vi "Q2.vi"() -> ()   [LabVIEW 2019]
uses:
  <vilib>/measure/matone.llb/Extract Multiple Tone Information N Chan.vi
  <vilib>/measure/NI_MAPro.lvlib
panel:
  in  "Boolean":bool
  out "Potência Ativa":i32
  out "multiple tone information":T1(array[cluster]) {"multiple tone information"."detected phase (deg)" format="%_6g"; "multiple tone information"."detected amplitude" format="%_6p"; "multiple tone information"."detected frequency" format="%_6p"}
  out "Waveform Graph":waveform(dbl)[](graph)
  in  "file path":path
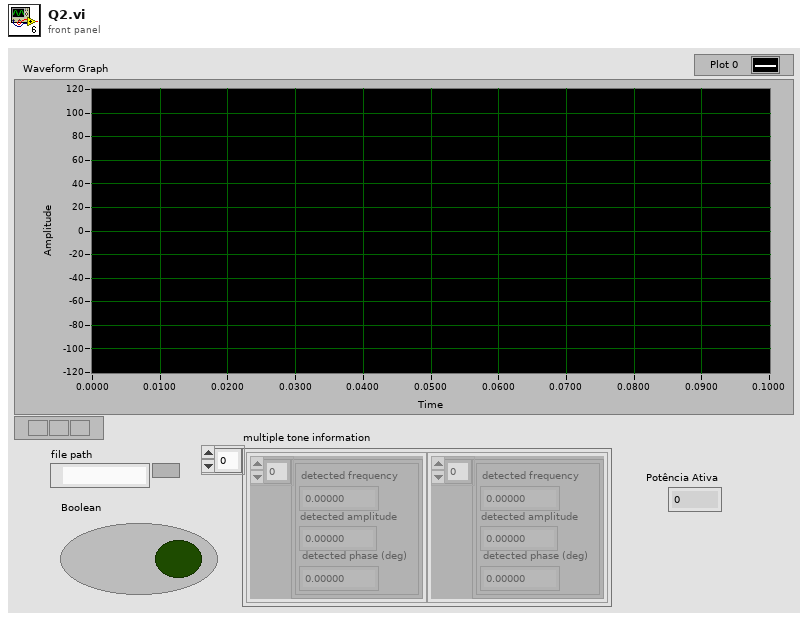
[diagram p1: front panel]
types:
  T1 = cluster{"multiple tone information":cluster{"detected frequency":dbl, "detected amplitude":dbl, "detected phase (deg)":dbl}[]}[]
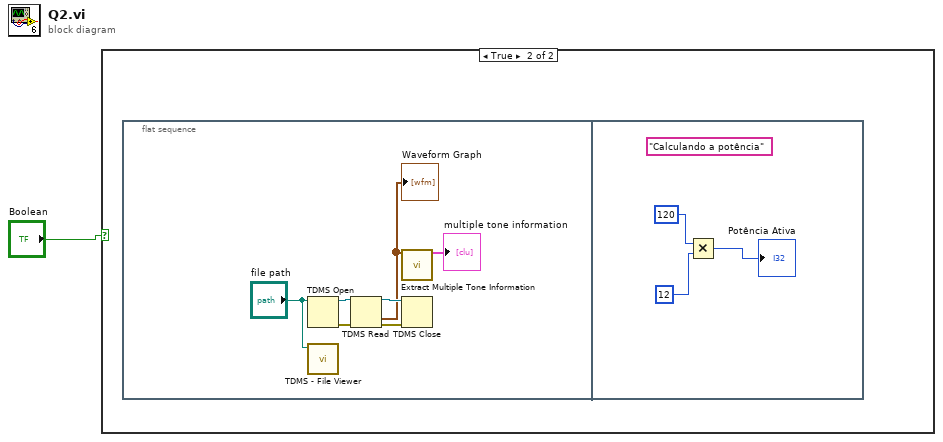
[diagram p0: block diagram]
diagram:
  n1 = case shown="True" "Boolean" {
    frame False {
    }
    frame True {
      n2 = flat-sequence {
        frame #0 {
          n3 = TDMS Open(11:"file path") -> (0:w7:errorcluster, 3:w8:refnum<k34>)  [unwired: 6 in]
          n4 = call <vilib>:"TDMS - File Viewer.vi"("file path"="file path") -> ()  [unwired: 5 in, 2 out]
          n5 = TDMS Read(0:w8, 11:w7) -> (4:w6:refnum<k34>, 10:w3:waveform(dbl)[], 15:w5:errorcluster)  [unwired: 6 in, 3 out]
          "Waveform Graph" <- w3
          n6 = call-poly <vilib>:"Extract Multiple Tone Information.vi"("time signals in"=w3) -> ("multiple tone information"=→"multiple tone information":T1)  [unwired: 12 in, 2 out]
          n7 = TDMS Close(8:w5, 11:w6) -> ()  [unwired: 2 out]
        }
        frame #1 {
          (unwired) "Calculando a potência"
          n8 = Multiply(x=120, y=12) -> (x*y=→"Potência Ativa":i32)
        }
      }
    }
  }
